vi "PID Integral Action Buffered (DBL Array).vi"(0 "previous output":dbl[](array[numeric]), 1 "previous error":dbl[](array[numeric]), 2 "PID Gains equal?":bool[](array[boolean]), 3 "previous integrated error":dbl[](array[numeric]), 4 "previous derivative action":dbl[](array[numeric]) format="%.2f", 5 "dt (min)":dbl format="%.3f", 6 "Ki":dbl[](array[numeric]) format="%.2f", 7 "initialize (F)":bool, 8 "proportional action":dbl[](array[numeric]) format="%.2f", 9 "linearity ([1])":dbl[](array[numeric]) format="%.2f", 10 "error":dbl[](array[numeric]) format="%.2f", 11 "auto? (T)":bool[](array[boolean]), 12 "output range":cluster{"output high":dbl, "output low":dbl}[](array[cluster]) {"output low" format="%.2f"; "output high" format="%.2f"}, 13 "manual control":dbl[](array[numeric])=[0.0] format="%.2f") -> (14 "output":dbl[](array[numeric]) format="%.2f", 17 "integrated error out":dbl[](array[numeric]))   [LabVIEW 2020, in "NI_PID_pid.lvlib"]
uses:
  NI_PID_pid.lvlib
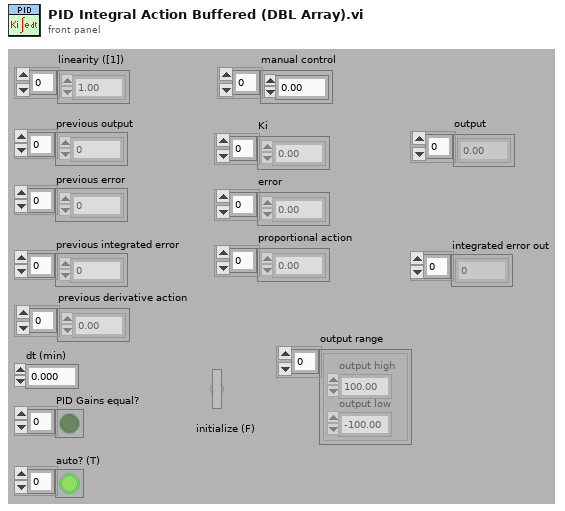
[diagram p1: front panel]
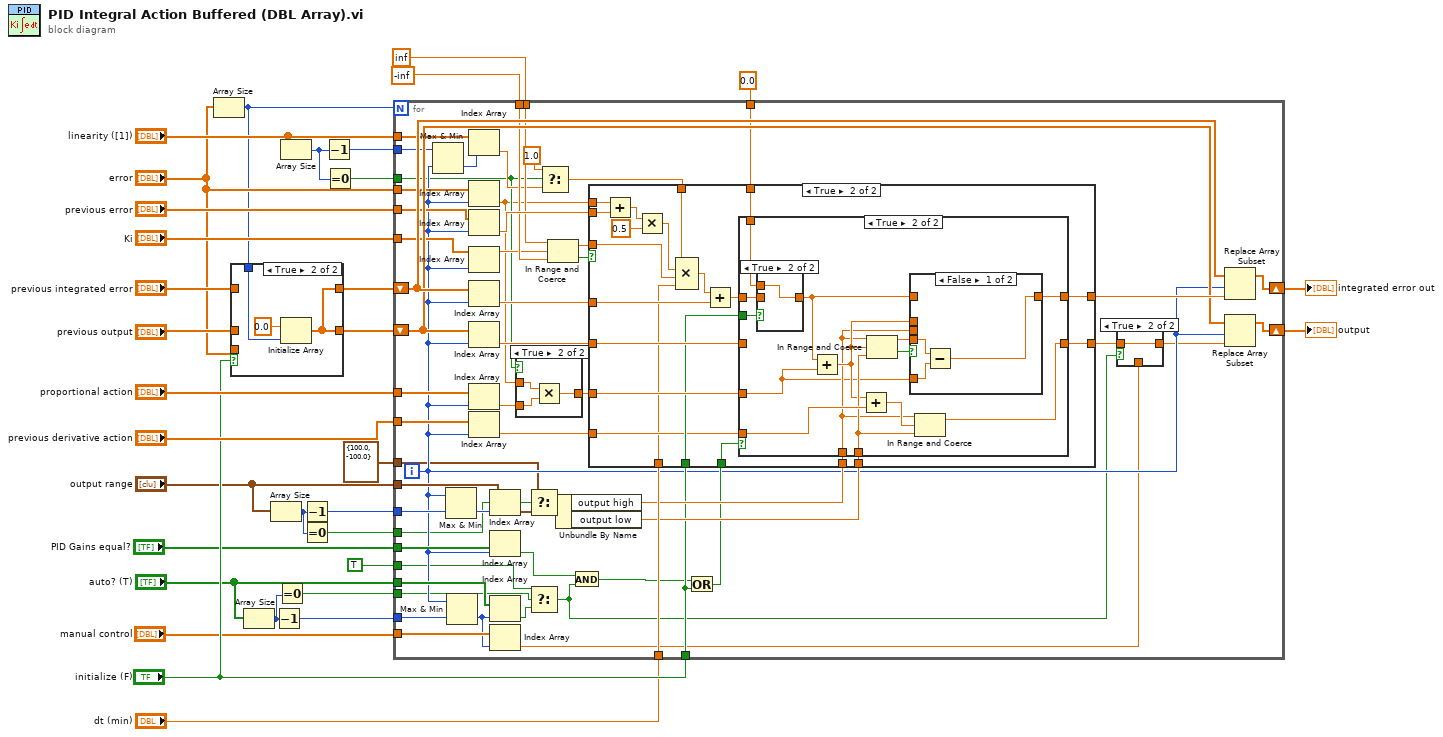
[diagram p0: block diagram]
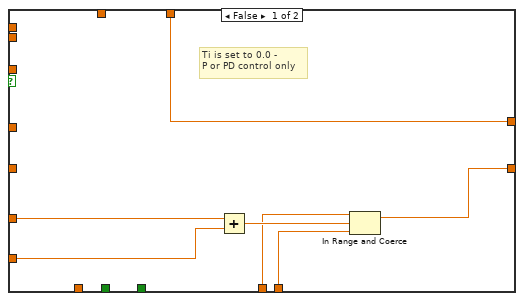
[diagram p5: hidden frame]
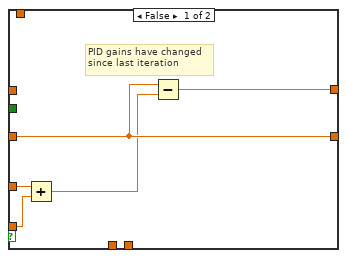
[diagram p6: hidden frame]
diagram:
  n1 = Array Size(array="error") -> (size(s)=w13:i32)
  n2 = case shown="True" "initialize (F)" {
    tunnel: "previous output" -> [w35 _]
    tunnel: [w35 w37] -> w26
    tunnel: "previous integrated error" -> [w34 _]
    tunnel: [w34 w37] -> w27
    tunnel: "error" -> [_ _]
    tunnel: w13 -> [_ w36]
    frame False {
    }
    frame True {
      n3 = Initialize Array(0.0 ("element"), w36) -> (w37:dbl[])
    }
  }
  n4 = Array Size(array="auto? (T)") -> (size(s)=w8:i32)
  n5 = Array Size(array="output range") -> (size(s)=w3:i32)
  n6 = Decrement(x=w8) -> (x-1=w10:i32)
  n7 = Equal To 0?(x=w8) -> (x = 0?=w7:bool)
  n8 = Array Size(array="linearity ([1])") -> (size(s)=w5:i32)
  n9 = Decrement(x=w3) -> (x-1=w12:i32)
  n10 = Equal To 0?(x=w3) -> (x = 0?=w2:bool)
  n11 = Decrement(x=w5) -> (x-1=w17:i32)
  n12 = Equal To 0?(x=w5) -> (x = 0?=w4:bool)
  n13 = for {
    N: w13 -> [_]
    tunnel: "previous error" -> [w83]
    tunnel: "proportional action" -> [w88]
    tunnel: "error" -> [w84]
    tunnel: "initialize (F)" -> [w62]
    tunnel: "PID Gains equal?" -> [w69]
    tunnel: "output range" -> [w68]
    tunnel: "previous derivative action" -> [w87]
    shift-right: [w91] -> w32
    shift-left: w27 -> [w93]
    shift-right: [w89] -> w30
    shift-left: w26 -> [w90]
    tunnel: "dt (min)" -> [w85]
    tunnel: "Ki" -> [w81]
    tunnel: inf ("upper limit") -> [w78]
    tunnel: -inf ("lower limit") -> [w77]
    tunnel: 0.0 ("t") -> [w76]
    tunnel: "linearity ([1])" -> [w72]
    tunnel: w17 -> [w71]
    tunnel: w12 -> [w67]
    tunnel: "auto? (T)" -> [w65]
    tunnel: w10 -> [w64]
    tunnel: "manual control" -> [w56]
    tunnel: w7 -> [w52]
    tunnel: TRUE ("t") -> [w51]
    tunnel: w4 -> [w42]
    tunnel: w2 -> [w46]
    tunnel: cluster{"output high":dbl, "output low":dbl} {"output high"=100.0, "output low"=-100.0} ("element") -> [w44]
    i -> [w59]
    n14 = Max & Min(x=w71, y=w59) -> (min(x,y)=w70:i32)  [unwired: 1 out]
    n15 = Max & Min(x=w59, y=w67) -> (min(x,y)=w66:i32)  [unwired: 1 out]
    n16 = Max & Min(x=w59, y=w64) -> (min(x,y)=w55:i32)  [unwired: 1 out]
    n17 = Index Array(array=w72, index=w70) -> (element=w48:dbl)
    n18 = Index Array(array=w84, index=w59) -> (element=w40:dbl)
    n19 = Index Array(array=w83, index=w59) -> (element=w82:dbl)
    n20 = Index Array(array=w81, index=w59) -> (element=w73:dbl)
    n21 = Index Array(array=w93, index=w59) -> (element=w94:dbl)
    n22 = Index Array(array=w90, index=w59) -> (element=w95:dbl)
    n23 = Index Array(array=w88, index=w59) -> (element=w41:dbl)
    n24 = Index Array(array=w87, index=w59) -> (element=w86:dbl)
    n25 = Index Array(array=w68, index=w66) -> (element=w45:cluster{"output high":dbl, "output low":dbl})
    n26 = Index Array(array=w69, index=w59) -> (element=w63:bool)
    n27 = Index Array(array=w65, index=w55) -> (element=w53:bool)
    n28 = Index Array(array=w56, index=w55) -> (element=w54:dbl)
    n29 = case shown="True" w42 {
      tunnel: w41 -> [w96 w98]
      tunnel: w40 -> [_ w99]
      tunnel: [w96 w97] -> w39
      frame False {
      }
      frame True {
        n30 = Multiply(x=w99, y=w98) -> (x*y=w97:dbl)
      }
    }
    n31 = Select(t=w44, s=w46, f=w45) -> (s? t:f=w43:cluster{"output high":dbl, "output low":dbl})
    n32 = Select(t=w51, s=w52, f=w53) -> (s? t:f=w50:bool)
    n33 = Select(t=1.0 ("f"), s=w42, f=w48) -> (s? t:f=w49:dbl)
    n34 = In Range and Coerce(upper limit=w78, x=w73, lower limit=w77) -> (coerced(x)=w80:dbl, In Range?=w79:bool)
    n35 = Unbundle By Name(w43) -> ("output high"=w75:dbl, "output low"=w74:dbl)
    n36 = And(x=w63, y=w50) -> (x .and. y?=w61:bool)
    n37 = Or(x=w61, y=w62) -> (x .or. y?=w60:bool)
    n38 = case shown="True" w79 {
      tunnel: w40 -> [_ w128]
      tunnel: w82 -> [_ w129]
      tunnel: w94 -> [_ w123]
      tunnel: [w104 w119] -> w92
      tunnel: w80 -> [_ w117]
      tunnel: w39 -> [w106 w121]
      tunnel: [w108 w118] -> w58
      tunnel: w95 -> [_ w120]
      tunnel: w62 -> [_ w116]
      tunnel: w60 -> [_ w115]
      tunnel: w86 -> [w107 w114]
      tunnel: w85 -> [_ w113]
      tunnel: w76 -> [w104 w112]
      tunnel: w75 -> [w102 w111]
      tunnel: w74 -> [w103 w110]
      tunnel: w49 -> [_ w109]
      frame False {
        # "Ti is set to 0.0 -\nP or PD control only"
        n39 = Add(x=w106, y=w107) -> (x+y=w105:dbl)
        n40 = In Range and Coerce(upper limit=w102, x=w105, lower limit=w103) -> (coerced(x)=w108:dbl)  [unwired: 1 out]
      }
      frame True {
        n41 = Add(x=w128, y=w129) -> (x+y=w126:dbl)
        n42 = Multiply(x=w126, y=0.5) -> (x*y=w125:dbl)
        n43 = Compound Arithmetic op=MULTIPLY(w109, w125, w117, w113) -> (w124:dbl)
        n44 = Add(x=w124, y=w123) -> (x+y=w122:dbl)
        n45 = case shown="True" w115 {
          tunnel: w122 -> [_ w143]
          tunnel: w121 -> [w131 w135]
          tunnel: w120 -> [w134 _]
          tunnel: w116 -> [_ w142]
          tunnel: [w133 w140] -> w119
          tunnel: [w134 w146] -> w118
          tunnel: w114 -> [w132 w147]
          tunnel: w112 -> [_ w144]
          tunnel: w111 -> [_ w136]
          tunnel: w110 -> [_ w145]
          frame False {
            # "PID gains have changed\nsince last iteration"
            n46 = Add(x=w131, y=w132) -> (x+y=w130:dbl)
            n47 = Subtract(x=w134, y=w130) -> (x-y=w133:dbl)
          }
          frame True {
            n48 = case shown="True" w142 {
              tunnel: w144 -> [_ w154]
              tunnel: [w153 w154] -> w141
              tunnel: w143 -> [w153 _]
              frame False {
              }
              frame True {
              }
            }
            n49 = Add(x=w141, y=w135) -> (x+y=w137:dbl)
            n50 = Add(x=w137, y=w147) -> (x+y=w148:dbl)
            n51 = In Range and Coerce(upper limit=w136, x=w137, lower limit=w145) -> (coerced(x)=w138:dbl, In Range?=w139:bool)
            n52 = case shown="False" w139 {
              tunnel: w141 -> [_ w152]
              tunnel: [w149 w152] -> w140
              tunnel: w138 -> [w151 _]
              tunnel: w135 -> [w150 _]
              tunnel: w136 -> [_ _]
              tunnel: w137 -> [_ _]
              frame False {
                n53 = Subtract(x=w151, y=w150) -> (x-y=w149:dbl)
              }
              frame True {
              }
            }
            n54 = In Range and Coerce(upper limit=w136, x=w148, lower limit=w145) -> (coerced(x)=w146:dbl)  [unwired: 1 out]
          }
        }
      }
    }
    n55 = case shown="True" w50 {
      tunnel: [w100 w101] -> w57
      tunnel: w58 -> [_ w101]
      tunnel: w54 -> [w100 _]
      frame False {
      }
      frame True {
      }
    }
    n56 = Replace Array Subset(array=w93, new element=w92, index=w59) -> (w91:dbl[])
    n57 = Replace Array Subset(array=w90, new element=w57, index=w59) -> (w89:dbl[])
  }
  "integrated error out" <- w32
  "output" <- w30
